vi "EEPROM烧录模块.vi"(8 "input_array_temp_int":u8[][](array[numeric]) format="%.0x", 9 "input_str_011string":string, 10 "Visa Port :":refnum<visa-resource-name>, 11 "Adaptor:":enum16{"RS232 - IIC", "LUXSHARE - IIC"}(ring)) -> (2 "show_str_coonmessage":string, 3 "show_bool_coon":bool)   [LabVIEW 2011]
uses:
  <vilib>/Utility/file.llb/Read From Spreadsheet File (string).vi
panel:
  out "数组":bool[](array[boolean])
  in  "路径":path
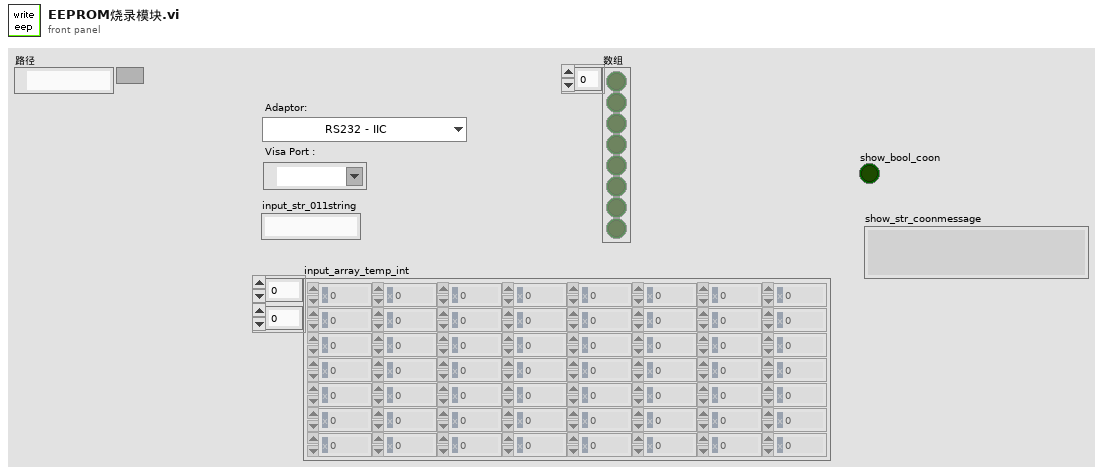
[diagram p1: front panel]
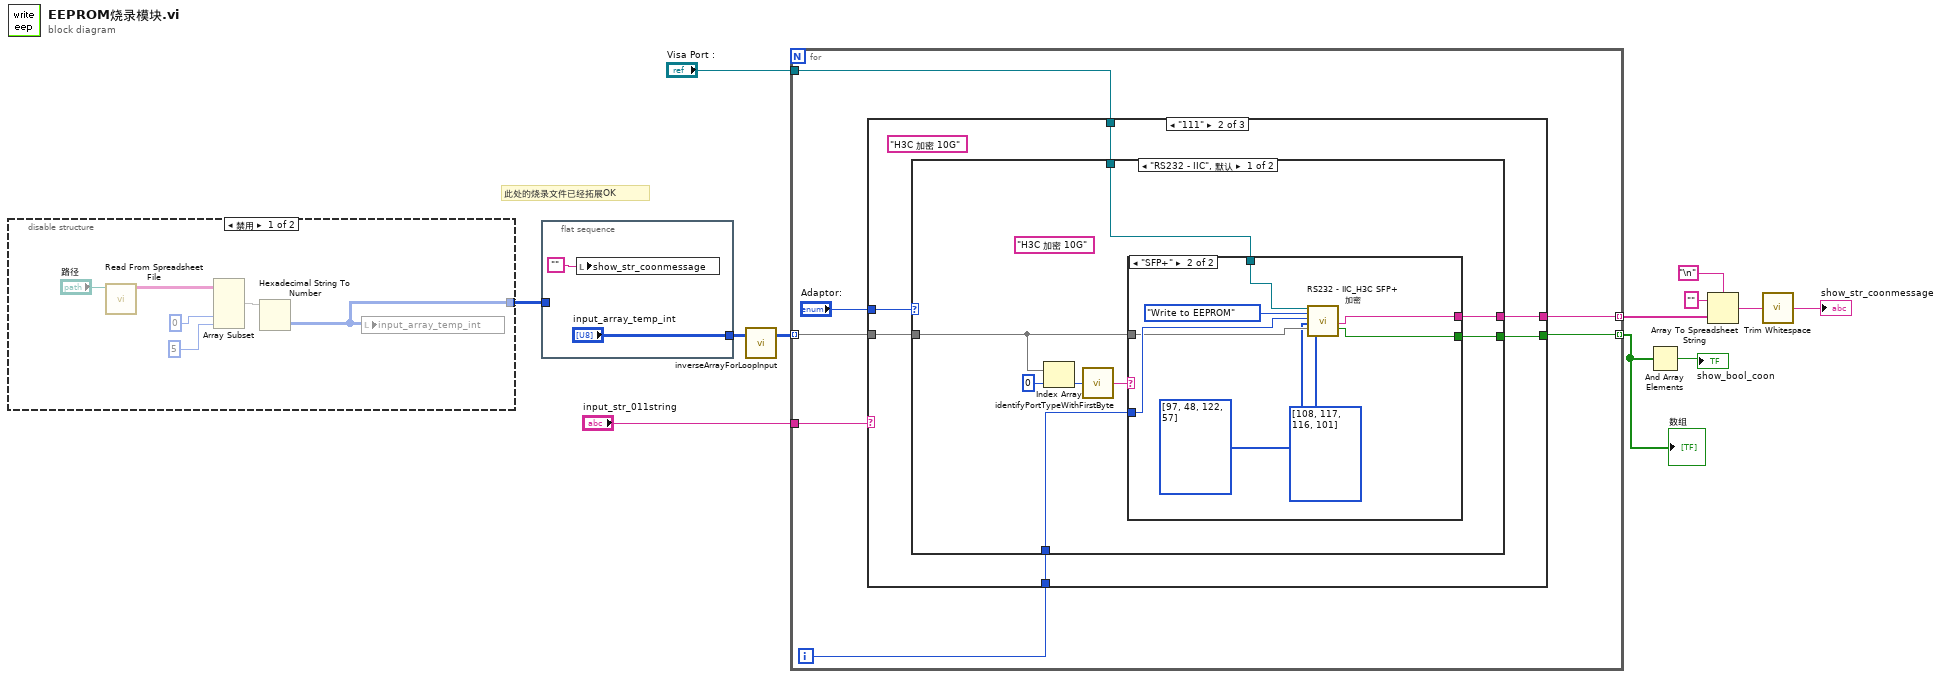
[diagram p0: block diagram]
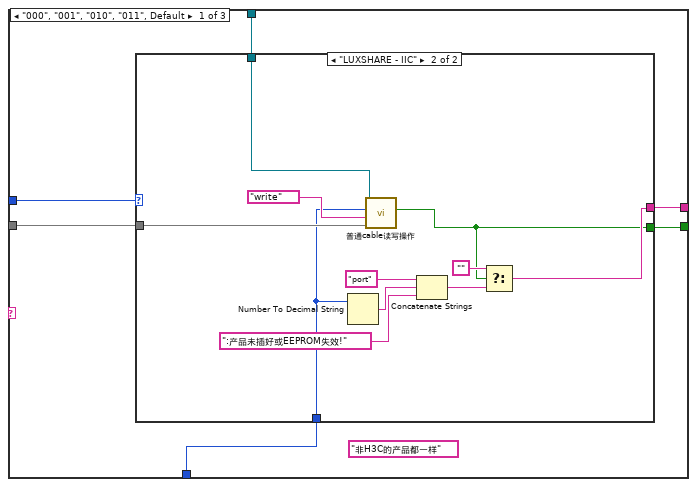
[diagram p3: hidden frame]
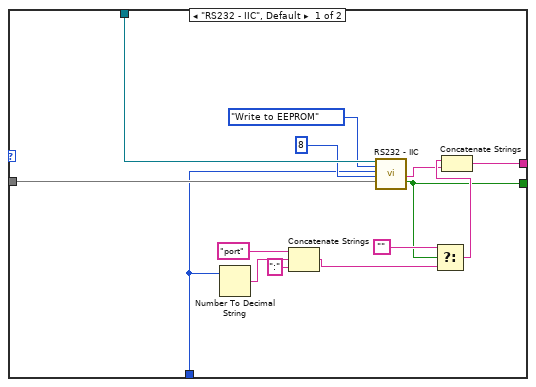
[diagram p4: hidden frame]
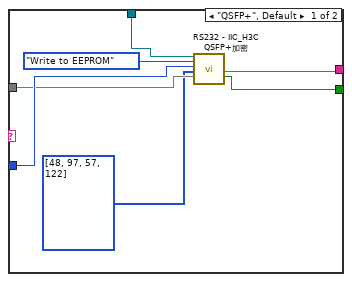
[diagram p5: hidden frame]
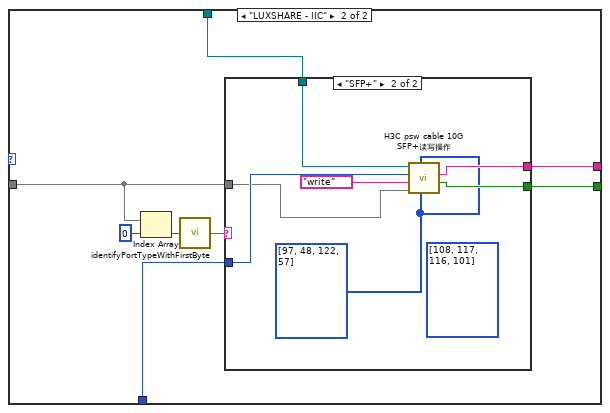
[diagram p6: hidden frame]
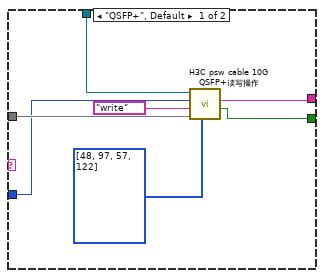
[diagram p7: hidden frame]
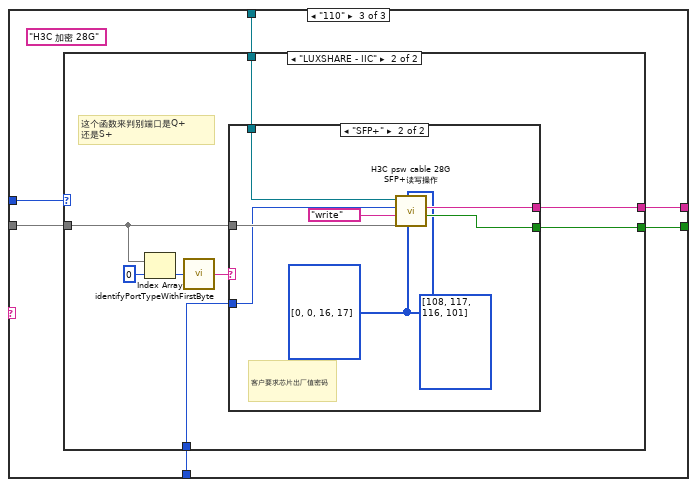
[diagram p8: hidden frame]
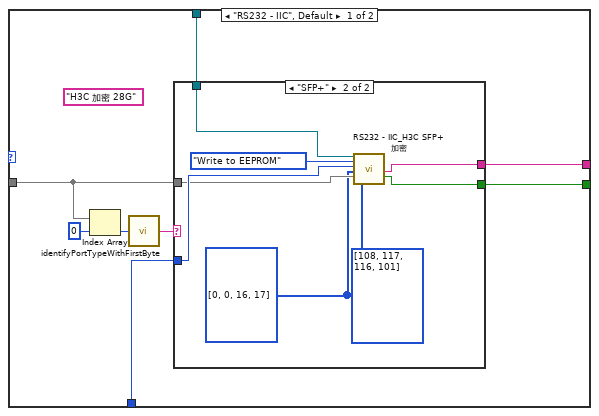
[diagram p9: hidden frame]
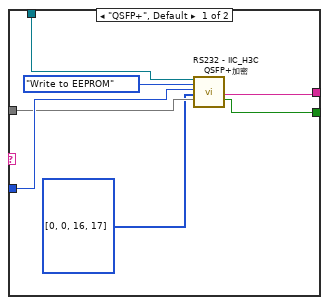
[diagram p10: hidden frame]
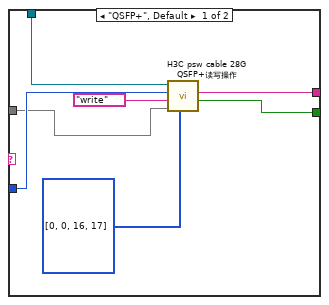
[diagram p11: hidden frame]
diagram:
  # "此处的烧录文件已经拓展OK"
  n1 = disable-structure shown="禁用" {
    disable-tunnel: [w13 _] -> w1
    frame Disabled {
      n2 = call-poly <vilib>:"Read From Spreadsheet File.vi"("file path (dialog if empty)"="路径") -> ("all rows"=w17:string[][])  [unwired: 6 in, 4 out]
      n3 = Array Subset(array=w17, index (col)=0 ("禁用的索引 (列)"), length (col)=5 ("长度")) -> (w16:string[][])  [unwired: 2 in]
      n4 = Hexadecimal String To Number(string=w16) -> (number=w13:u32[][])  [unwired: 2 in, 1 out]
      n5 = local write "input_array_temp_int"(w13) -> ()
    }
    frame Enabled {
    }
  }
  n6 = flat-sequence {
    tunnel: ["input_array_temp_int"] -> w9
    tunnel: w1 -> [_]
    frame #0 {
      n7 = local write "show_str_coonmessage"("") -> ()
    }
  }
  n8 = call "inverseArrayForLoopInput.vi"("input_array_temp_int"=w9) -> ("show_array_temp_int"=w10:u8[][])  [unwired: 1 in, 1 out]
  n9 = for {
    tunnel: "Visa Port :" -> [w27]
    tunnel: w10 -> [w25] mode=indexing
    tunnel: [w24] -> w3 mode=indexing
    tunnel: [w23] -> w8 mode=indexing
    tunnel: "input_str_011string" -> [w22]
    i -> [w26]
    n10 = case shown="\"111\"" w22 {
      tunnel: w27 -> [w33 w64 w114]
      tunnel: w25 -> [w32 w62 w112]
      tunnel: w26 -> [w31 w63 w113]
      tunnel: [w30 w61 w111] -> w23
      tunnel: [w29 w60 w110] -> w24
      tunnel: "Adaptor:" -> [w28 w59 w109]
      frame "000", "001", "010", "011", Default {
        (unwired) "非H3C的产品都一样"
        n11 = case shown="\"LUXSHARE - IIC\"" w28 {
          tunnel: w33 -> [w47 w58]
          tunnel: w32 -> [w45 w56]
          tunnel: w31 -> [w42 w50]
          tunnel: [w38 w49] -> w30
          tunnel: [w34 w48] -> w29
          frame "RS232 - IIC", Default {
            n12 = Number To Decimal String(number=w42) -> (decimal integer string=w41:string)  [unwired: 1 in]
            n13 = Concatenate Strings("port", w41, ":" ("字符串")) -> (w37:string)
            n14 = call "RS232 - IIC.vi"("VISA resource name"=w47, "Function"=enum16{"Write to EEPROM", "Read From EEPROM"}."Write to EEPROM", "Select channel"=w42, "WData size"=u32 8, "Data to write"=w45) -> ("Message"=w35:string, "Result"=w34:bool)  [unwired: 8 in, 5 out]
            n15 = Select(t="", s=w34, f=w37) -> (s? t:f=w36:string)
            n16 = Concatenate Strings(w36, w35) -> (w38:string)
          }
          frame "LUXSHARE - IIC" {
            n17 = Number To Decimal String(number=w50) -> (decimal integer string=w54:string)  [unwired: 1 in]
            n18 = call "普通cable读写操作.vi"("input_data"=w56, "input_mode"="write", "Channel"=w50, "VISA"=w58) -> ("result"=w48:bool)  [unwired: 6 in, 1 out]
            n19 = Concatenate Strings("port", w54, ":产品未插好或EEPROM失效!" ("字符串")) -> (w51:string)
            n20 = Select(t="", s=w48, f=w51) -> (s? t:f=w49:string)
          }
        }
      }
      frame "111" {
        (unwired) "H3C 加密 10G"
        n21 = case shown="\"RS232 - IIC\", 默认" w59 {
          tunnel: w64 -> [w69 w91]
          tunnel: w63 -> [w68 w90]
          tunnel: w62 -> [w67 w89]
          tunnel: [w66 w88] -> w61
          tunnel: [w65 w87] -> w60
          frame "RS232 - IIC", Default {
            (unwired) "H3C 加密 10G"
            n22 = Index Array(array=w67, index=0 ("索引")) -> (element=w71:u8)
            n23 = call "identifyPortTypeWithFirstByte.vi"("input_int"=w71) -> ("show_str_portType"=w70:string)
            n24 = case shown="\"SFP+\"" w70 {
              tunnel: w69 -> [w79 w86]
              tunnel: w68 -> [w77 w84]
              tunnel: w67 -> [w76 w83]
              tunnel: [w75 w82] -> w65
              tunnel: [w74 w81] -> w66
              frame "QSFP+", Default {
                n25 = call "RS232 - IIC_H3C QSFP+加密.vi"("VISA resource name"=w79, "Function"=enum16{"Write to EEPROM", "Read From EEPROM"}."Write to EEPROM", "Select channel"=w77, "input_psw"=u8[] [48, 97, 57, 122], "Data to write"=w76) -> ("Message"=w74:string, "status"=w75:bool)  [unwired: 7 in, 6 out]
              }
              frame "SFP+" {
                (unwired) u8[] [108, 117, 116, 101]
                w80 = u8[] [97, 48, 122, 57]
                n26 = call "RS232 - IIC_H3C SFP+ 加密.vi"("VISA resource name"=w86, "Function"=enum16{"Write to EEPROM", "Read From EEPROM"}."Write to EEPROM", "Select channel"=w84, "psw"=w80, "Data to write"=w83, "psw 2"=w80) -> ("Message"=w81:string, "state"=w82:bool)  [unwired: 7 in, 5 out]
              }
            }
          }
          frame "LUXSHARE - IIC" {
            n27 = Index Array(array=w89, index=0 ("索引")) -> (element=w93:u8)
            n28 = call "identifyPortTypeWithFirstByte.vi"("input_int"=w93) -> ("show_str_portType"=w92:string)
            n29 = case shown="\"SFP+\"" w92 {
              tunnel: w91 -> [w101 w108]
              tunnel: w90 -> [w99 w107]
              tunnel: w89 -> [w100 w105]
              tunnel: [w95 w103] -> w87
              tunnel: [w96 w104] -> w88
              frame "QSFP+", Default {
                n30 = call "H3C psw cable 10G QSFP+读写操作.vi"("input_psw"=u8[] [48, 97, 57, 122], "input_data"=w100, "input_mode"="write", "Channel"=w99, "VISA"=w101) -> ("result"=w95:bool, "message"=w96:string)  [unwired: 3 in, 2 out]
              }
              frame "SFP+" {
                (unwired) u8[] [108, 117, 116, 101]
                w102 = u8[] [97, 48, 122, 57]
                n31 = call "H3C psw cable 10G SFP+读写操作.vi"("input_psw"=w102, "input_psw 2"=w102, "input_data"=w105, "input_mode"="write", "Channel"=w107, "VISA"=w108) -> ("result"=w103:bool, "message"=w104:string)  [unwired: 2 in, 2 out]
              }
            }
          }
        }
      }
      frame "110" {
        (unwired) "H3C 加密 28G"
        n32 = case shown="\"LUXSHARE - IIC\"" w109 {
          tunnel: w114 -> [w119 w141]
          tunnel: w113 -> [w118 w140]
          tunnel: w112 -> [w117 w139]
          tunnel: [w116 w138] -> w111
          tunnel: [w115 w137] -> w110
          frame "RS232 - IIC", Default {
            (unwired) "H3C 加密 28G"
            n33 = Index Array(array=w117, index=0 ("索引")) -> (element=w121:u8)
            n34 = call "identifyPortTypeWithFirstByte.vi"("input_int"=w121) -> ("show_str_portType"=w120:string)
            n35 = case shown="\"SFP+\"" w120 {
              tunnel: w119 -> [w129 w136]
              tunnel: w118 -> [w127 w134]
              tunnel: w117 -> [w126 w133]
              tunnel: [w125 w132] -> w115
              tunnel: [w124 w131] -> w116
              frame "QSFP+", Default {
                n36 = call "RS232 - IIC_H3C QSFP+加密.vi"("VISA resource name"=w129, "Function"=enum16{"Write to EEPROM", "Read From EEPROM"}."Write to EEPROM", "Select channel"=w127, "input_psw"=u8[] [0, 0, 16, 17], "Data to write"=w126) -> ("Message"=w124:string, "status"=w125:bool)  [unwired: 7 in, 6 out]
              }
              frame "SFP+" {
                (unwired) u8[] [108, 117, 116, 101]
                w130 = u8[] [0, 0, 16, 17]
                n37 = call "RS232 - IIC_H3C SFP+ 加密.vi"("VISA resource name"=w136, "Function"=enum16{"Write to EEPROM", "Read From EEPROM"}."Write to EEPROM", "Select channel"=w134, "psw"=w130, "Data to write"=w133, "psw 2"=w130) -> ("Message"=w131:string, "state"=w132:bool)  [unwired: 7 in, 5 out]
              }
            }
          }
          frame "LUXSHARE - IIC" {
            # "这个函数来判别端口是Q+\n还是S+"
            n38 = Index Array(array=w139, index=0 ("索引")) -> (element=w143:u8)
            n39 = call "identifyPortTypeWithFirstByte.vi"("input_int"=w143) -> ("show_str_portType"=w142:string)
            n40 = case shown="\"SFP+\"" w142 {
              tunnel: w141 -> [w151 w156]
              tunnel: w140 -> [w150 w154]
              tunnel: w139 -> [w145 w155]
              tunnel: [w147 w157] -> w137
              tunnel: [w148 w158] -> w138
              frame "QSFP+", Default {
                n41 = call "H3C psw cable 28G QSFP+读写操作.vi"("input_psw"=u8[] [0, 0, 16, 17], "input_data"=w145, "input_mode"="write", "Channel"=w150, "VISA"=w151) -> ("result"=w147:bool, "message"=w148:string)  [unwired: 3 in, 2 out]
              }
              frame "SFP+" {
                (unwired) u8[] [108, 117, 116, 101]
                w152 = u8[] [0, 0, 16, 17]
                # "客户要求芯片出厂值密码"
                n42 = call "H3C psw cable 28G SFP+读写操作.vi"("input_psw"=w152, "input_psw 2"=w152, "input_data"=w155, "input_mode"="write", "Channel"=w154, "VISA"=w156) -> ("result"=w157:bool, "message"=w158:string)  [unwired: 2 in, 2 out]
              }
            }
          }
        }
      }
    }
  }
  "数组" <- w3
  n43 = And Array Elements(Boolean array=w3) -> (logical AND=→"show_bool_coon":bool)
  n44 = Array To Spreadsheet String(delimiter (Tab)="\n" ("分隔符(Tab)"), array=w8, 3:"" ("格式字符串")) -> (spreadsheet string=w5:string)
  n45 = call <vilib>:"Trim Whitespace.vi"("string"=w5) -> ("trimmed string"=→"show_str_coonmessage":string)  [unwired: 1 in]
